vi "Image_Snap.vi"(6 "Crop?":bool, 8 "error in":errorcluster, 9 "Enum":T1, 11 "input cluster":T3={"L16 Linear Actuator"="", "XE 1000 Pump"="", "Camera1"="", "Camera2"="", "Camera1_IMG"=refnum, "Camera2_IMG"=refnum, "Img_Capt"=FALSE, "Actuator"=FALSE, "Pump"=FALSE, "Cam 1"=FALSE, "Cam 2"=FALSE, "Empty_Refill"=FALSE, "Crop"=FALSE, "Period"=0, "Light intensity"=100, "Exposure Time"=1000.0} {"Light intensity" scale=0.0..100.0}) -> (0 "error out":errorcluster, 3 "Image Out":T2)   [LabVIEW 2019]
uses:
  controls/Data.ctl
  <vilib>/userdefined/High Color/IMAQdx.ctl
  <vilib>/vision/Image Controls.llb/IMAQ Image.ctl
  Camera_ID.ctl
  <vilib>/vision/driver/NI_Vision_Acquisition_Software.lvlib
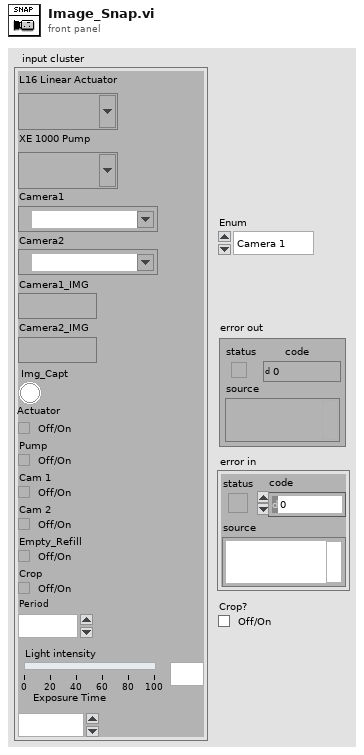
[diagram p1: front panel]
types:
  T1 = typedef "Camera_ID.ctl" = enum16{"Camera 1", "Camera 2"}
  T2 = typedef "IMAQ Image.ctl" = refnum<image>
  T3 = typedef "Data.ctl" = cluster{"L16 Linear Actuator":refnum<visa-resource-name>, "XE 1000 Pump":refnum<visa-resource-name>, "Camera1":T4, "Camera2":T4, "Camera1_IMG":T2, "Camera2_IMG":T2, "Img_Capt":bool, "Actuator":bool, "Pump":bool, "Cam 1":bool, "Cam 2":bool, "Empty_Refill":bool, "Crop":bool, "Period":i64, "Light intensity":i32, "Exposure Time":dbl}
  T4 = typedef "IMAQdx.ctl" = refnum<k21>
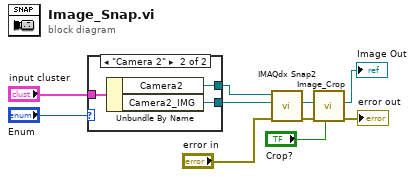
[diagram p0: block diagram]
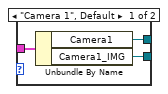
[diagram p2: hidden frame]
diagram:
  n1 = case shown="\"Camera 2\"" "Enum" {
    tunnel: "input cluster" -> [w13 w14]
    tunnel: [w12 w16] -> w9
    tunnel: [w11 w15] -> w8
    frame "Camera 1", Default {
      n2 = Unbundle By Name(w13) -> ("Camera1"=w12:T4, "Camera1_IMG"=w11:T2)
    }
    frame "Camera 2" {
      n3 = Unbundle By Name(w14) -> ("Camera2"=w16:T4, "Camera2_IMG"=w15:T2)
    }
  }
  n4 = call <vilib>:"IMAQdx Snap2.vi"("error in"="error in", "Image In"=w8, "Session In"=w9) -> ("error out"=w7:errorcluster, "Image Out"=w5:T2)  [unwired: 6 in, 1 out]
  n5 = call "Image_Crop.vi"("Crop?"="Crop?", "error in"=w7, "Image In"=w5) -> ("error out"=→"error out":errorcluster, "Image Out"=→"Image Out":T2)  [unwired: 7 in]
